vi "setMode.vi"(8 "error in (no error)":errorcluster, 10 "Mode":enum16{"Asynch Shutter", "Video"}(ring)=enum."Video", 11 "PixelflySettings in":refnum<class "PixelflySettings.lvclass">) -> (0 "error out":errorcluster, 3 "PixelflySettings out":refnum<class "PixelflySettings.lvclass">)   [LabVIEW 2011, in "Tools.lvlib" / "Settings.lvlib" / "PixelflySettings.lvclass"]
uses:
  PixelflySettings.lvclass
  PixelflySettings.lvclass/PixelflySettings.ctl
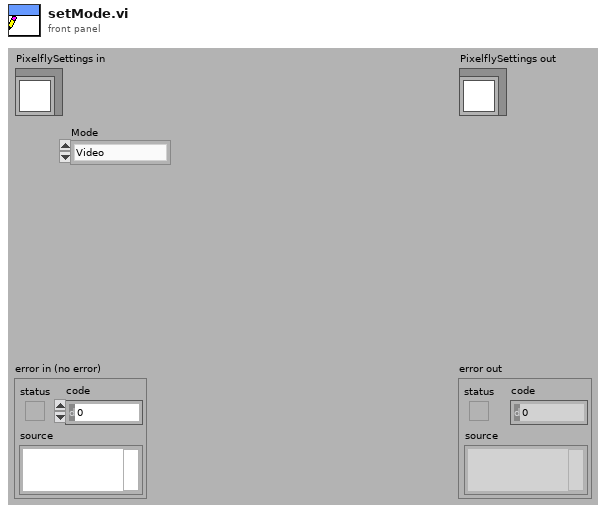
[diagram p1: front panel]
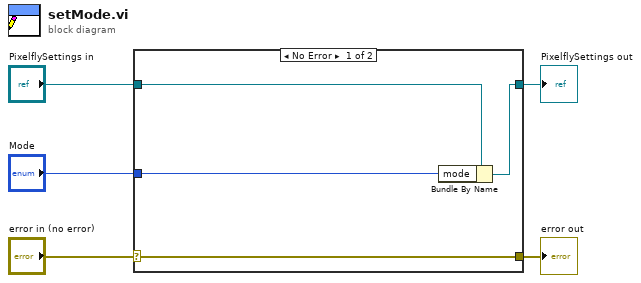
[diagram p0: block diagram]
diagram:
  n1 = case shown="No Error" "error in (no error)" {
    selector: "error in (no error)" -> [w9 w10]
    tunnel: [w9 w10] -> w4
    tunnel: [w7 w11] -> w2
    tunnel: "PixelflySettings in" -> [w8 w11]
    tunnel: "Mode" -> [w6 _]
    frame No Error {
      n2 = Bundle By Name(cluster=w8, "mode"=w6) -> (w7:refnum<class "PixelflySettings.lvclass">)
    }
    frame Error {
    }
  }
  "error out" <- w4
  "PixelflySettings out" <- w2
